vi "Configure Arming (External).vi"(0 "VISA resource name":refnum<visa-resource-name>, 1 "Measurement (0:Frequency)":i32(ring) items=["Frequency", "Frequency Ratio", "Period", "Totalize", "Phase", "Edge Rise Time", "Edge Fall Time", "Positive Pulse Width", "Negative Pulse Width", "Duty Cycle", "Time Interval", "Volt Maximum", "Volt Minimum"], 5 "Start Slope (0:Positive)":i32(ring) items=["Positive", "Negative"], 7 "Stop Type (0:Auto)":i32(ring) items=["Auto", "Positive", "Negative", "Time"], 9 "Stop Time (0.1s)":dbl=0.1 format="%^#_6g", 11 "error in (no error)":errorcluster, 12 "Time Interval Start":T1 {"Start Slope" items=["Positive", "Negative"]; "Start Delay Value" format="%^#_7g"; "Start Delay Type" items=["None", "Time", "Event"]}, 13 "Time Interval Stop":T2 {"Stop Delay Value" format="%^#_7g"; "Stop Delay Type" items=["None", "Time", "Event"]; "Stop Slope" items=["Positive", "Negative"]; "Stop Type" items=["Auto", "External"]}) -> (4 "VISA resource name out":refnum<visa-resource-name>, 15 "error out":errorcluster)   [LabVIEW 2013, in "Counter.lvlib" / "PICOTEST U62XXA series.lvlib"]
doc: "Configures the parameters required for External Arming. This VI should be called after the Configure Measurement VI.\n\n<B>Note:</B>\n\nVolt Peak Measurements <B>does not</B> have External Arming capabilities. Totalize Measurement <B>does not</B> support Auto stop type. The <B>clusters</B> are for Time Interval Measurement only."
uses:
  PICOTEST U62XXA series.lvlib
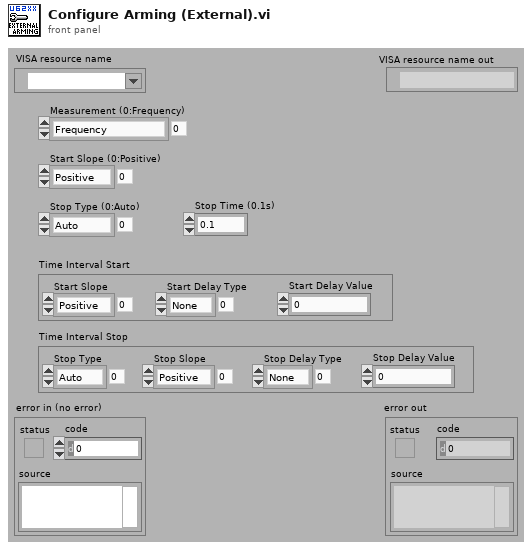
[diagram p1: front panel]
types:
  T1 = cluster{"Start Delay Type":i32, "Start Delay Value":dbl, "Start Slope":i32}
  T2 = cluster{"Stop Type":i32, "Stop Slope":i32, "Stop Delay Type":i32, "Stop Delay Value":dbl}
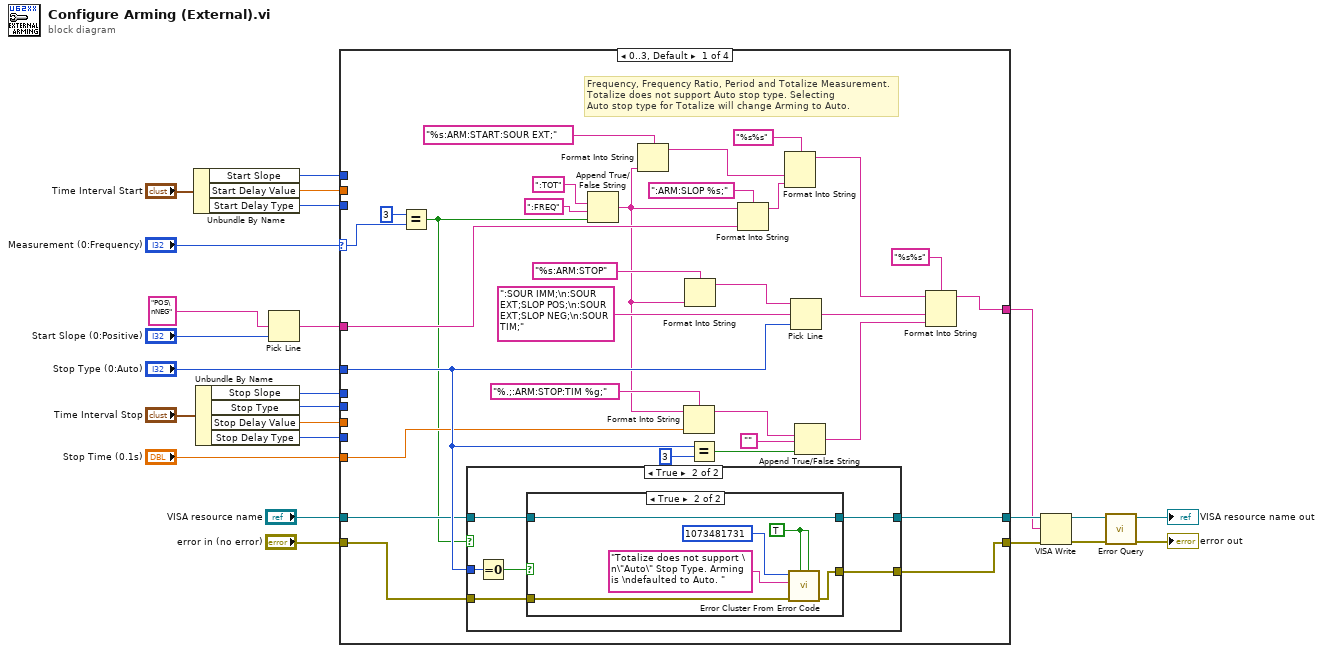
[diagram p0: block diagram]
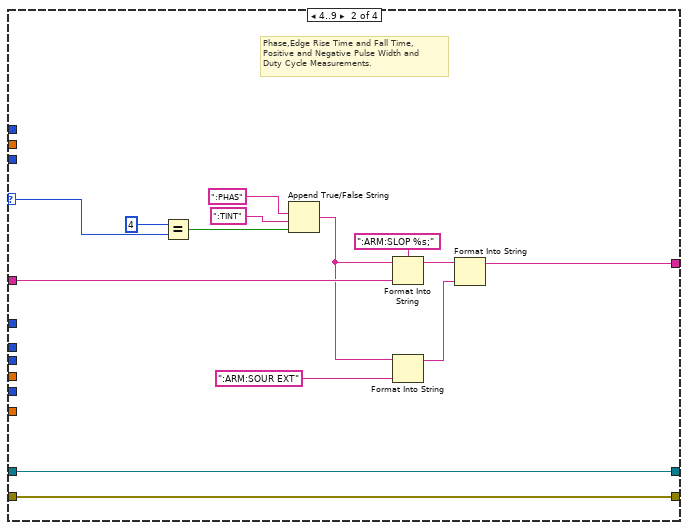
[diagram p4: hidden frame]
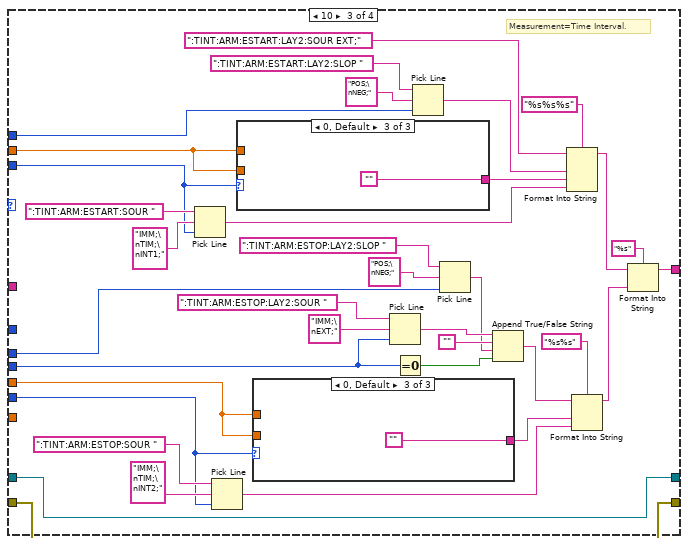
[diagram p5: hidden frame]
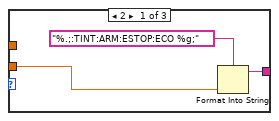
[diagram p6: hidden frame]
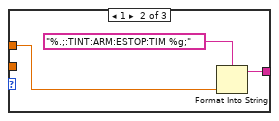
[diagram p7: hidden frame]
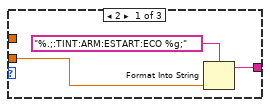
[diagram p8: hidden frame]
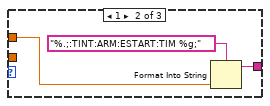
[diagram p9: hidden frame]
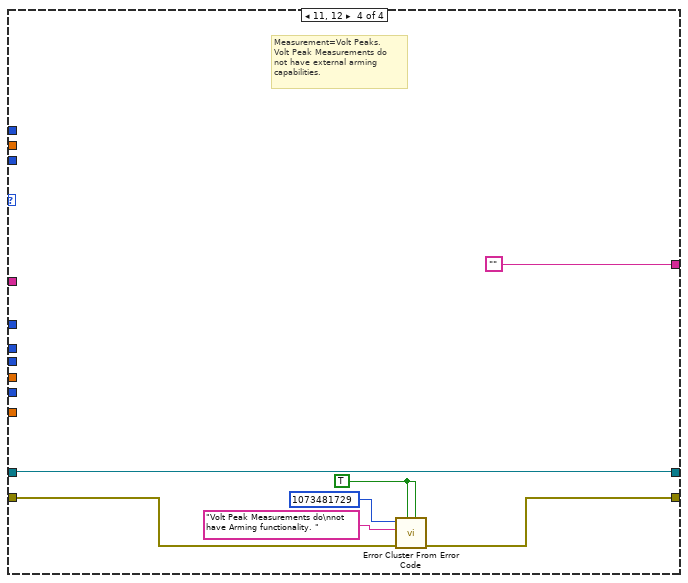
[diagram p10: hidden frame]
diagram:
  n1 = Unbundle By Name("Time Interval Start") -> ("Start Slope"=w13:i32, "Start Delay Value"=w12:dbl, "Start Delay Type"=w11:i32)
  n2 = Unbundle By Name("Time Interval Stop") -> ("Stop Slope"=w9:i32, "Stop Type"=w6:i32, "Stop Delay Value"=w7:dbl, "Stop Delay Type"=w8:i32)
  n3 = Pick Line(multi-line string="POS\nNEG", line index="Start Slope (0:Positive)") -> (output string=w21:string)  [unwired: 1 in]
  n4 = case shown="0..3, Default" "Measurement (0:Frequency)" {
    selector: "Measurement (0:Frequency)" -> [w54 w84 _ _]
    tunnel: w21 -> [w52 w82 _ _]
    tunnel: [w28 w72 w89 ""] -> w1
    tunnel: "Stop Time (0.1s)" -> [w38 _ _ _]
    tunnel: "Stop Type (0:Auto)" -> [w43 _ _ _]
    tunnel: w13 -> [_ _ w112 _]
    tunnel: w12 -> [_ _ w111 _]
    tunnel: w11 -> [_ _ w110 _]
    tunnel: w9 -> [_ _ w103 _]
    tunnel: w6 -> [_ _ w102 _]
    tunnel: w8 -> [_ _ w109 _]
    tunnel: w7 -> [_ _ w108 _]
    tunnel: "VISA resource name" -> [w40 w78 w101 w138]
    tunnel: [w39 w78 w101 w138] -> w4
    tunnel: "error in (no error)" -> [w42 w77 w100 w139]
    tunnel: [w41 w77 w100 w137] -> w2
    frame 0..3, Default {
      # "Frequency, Frequency Ratio, Period and Totalize Measurement. \nTotalize does not support Auto stop type. Selecting\nAuto stop type for Totalize will change Arming to Auto."
      n5 = Equal?(x=3 ("y"), y=w54) -> (x = y?=w37:bool)
      n6 = case shown="True" w37 {
        tunnel: w43 -> [_ w62]
        tunnel: w42 -> [w56 w61]
        tunnel: [w56 w60] -> w41
        tunnel: w40 -> [w57 w59]
        tunnel: [w57 w58] -> w39
        frame False {
        }
        frame True {
          n7 = Equal To 0?(x=w62) -> (x = 0?=w63:bool)
          n8 = case shown="True" w63 {
            tunnel: w61 -> [w65 w68]
            tunnel: [w65 w67] -> w60
            tunnel: w59 -> [w64 w66]
            tunnel: [w64 w66] -> w58
            frame False {
            }
            frame True {
              w69 = TRUE ("is warning? (False)")
              n9 = call <vilib>:"Error Cluster From Error Code.vi"("is warning? (False)"=w69, "show call chain? (False)"=w69, "error in (no error)"=w68, "error message (\"\")"="Totalize does not support \n\"Auto\" Stop Type. Arming is \ndefaulted to Auto. " ("error message (\"\")"), "error code (0)"=1073481731 ("Code")) -> ("error out"=w67:errorcluster)  [unwired: 4 in]
            }
          }
        }
      }
      n10 = Append True/False String(1:w37, 2:":FREQ" ("multi-line string"), 3:":TOT" ("multi-line string")) -> (0:w31:string)  [unwired: 1 in]
      n11 = Format Into String(format string="%s:ARM:START:SOUR EXT;" ("multi-line string"), w31) -> (resulting string=w34:string)  [unwired: 2 in, 1 out]
      n12 = Format Into String(format string="%.;:ARM:STOP:TIM %g;", initial string=w31, w38) -> (resulting string=w47:string)  [unwired: 1 in, 1 out]
      n13 = Format Into String(format string="%s:ARM:STOP" ("multi-line string"), w31) -> (resulting string=w30:string)  [unwired: 2 in, 1 out]
      n14 = Equal?(x=w43, y=3) -> (x = y?=w48:bool)
      n15 = Format Into String(format string=":ARM:SLOP %s;", initial string=w31, w52) -> (resulting string=w33:string)  [unwired: 1 in, 1 out]
      n16 = Format Into String(format string="%s%s", w34, w33) -> (resulting string=w27:string)  [unwired: 2 in, 1 out]
      n17 = Pick Line(string ("")=w30, multi-line string=":SOUR IMM;\n:SOUR EXT;SLOP POS;\n:SOUR EXT;SLOP NEG;\n:SOUR TIM;", line index=w43) -> (output string=w26:string)
      n18 = Append True/False String(1:w48, 2:"", 3:w47) -> (0:w25:string)  [unwired: 1 in]
      n19 = Format Into String(format string="%s%s", initial string=w27, w26, w25) -> (resulting string=w28:string)  [unwired: 1 in, 1 out]
    }
    frame 4..9 {
      # "Phase,Edge Rise Time and Fall Time,\nPositive and Negative Pulse Width and\nDuty Cycle Measurements."
      n20 = Equal?(x=4 ("y"), y=w84) -> (x = y?=w79:bool)
      n21 = Append True/False String(1:w79, 2:":TINT" ("multi-line string"), 3:":PHAS" ("multi-line string")) -> (0:w76:string)  [unwired: 1 in]
      n22 = Format Into String(format string=":ARM:SLOP %s;", initial string=w76, w82) -> (resulting string=w74:string)  [unwired: 1 in, 1 out]
      n23 = Format Into String(initial string=w76, ":ARM:SOUR EXT" ("multi-line string")) -> (resulting string=w73:string)  [unwired: 2 in, 1 out]
      n24 = Format Into String(initial string=w74, w73) -> (resulting string=w72:string)  [unwired: 2 in, 1 out]
    }
    frame 10 {
      # "Measurement=Time Interval."
      n25 = Pick Line(string ("")=":TINT:ARM:ESTART:SOUR ", multi-line string="IMM;\nTIM;\nINT1;", line index=w110) -> (output string=w94:string)
      n26 = Pick Line(string ("")=":TINT:ARM:ESTOP:SOUR ", multi-line string="IMM;\nTIM;\nINT2;", line index=w109) -> (output string=w90:string)
      n27 = case shown="0, Default" w110 {
        tunnel: [w130 w133 ""] -> w95
        tunnel: w111 -> [w129 _ _]
        tunnel: w111 -> [_ w132 _]
        frame 2 {
          n28 = Format Into String(format string="%.;:TINT:ARM:ESTART:ECO %g;", w129) -> (resulting string=w130:string)  [unwired: 2 in, 1 out]
        }
        frame 1 {
          n29 = Format Into String(format string="%.;:TINT:ARM:ESTART:TIM %g;", w132) -> (resulting string=w133:string)  [unwired: 2 in, 1 out]
        }
        frame 0, Default {
        }
      }
      n30 = case shown="0, Default" w109 {
        tunnel: [w123 w126 ""] -> w91
        tunnel: w108 -> [_ w125 _]
        tunnel: w108 -> [w122 _ _]
        frame 2 {
          n31 = Format Into String(format string="%.;:TINT:ARM:ESTOP:ECO %g;", w122) -> (resulting string=w123:string)  [unwired: 2 in, 1 out]
        }
        frame 1 {
          n32 = Format Into String(format string="%.;:TINT:ARM:ESTOP:TIM %g;", w125) -> (resulting string=w126:string)  [unwired: 2 in, 1 out]
        }
        frame 0, Default {
        }
      }
      n33 = Pick Line(string ("")=":TINT:ARM:ESTOP:LAY2:SOUR ", multi-line string="IMM;\nEXT;", line index=w102) -> (output string=w107:string)
      n34 = Equal To 0?(x=w102) -> (x = 0?=w106:bool)
      n35 = Pick Line(string ("")=":TINT:ARM:ESTART:LAY2:SLOP ", multi-line string="POS;\nNEG;", line index=w112) -> (output string=w96:string)
      n36 = Pick Line(string ("")=":TINT:ARM:ESTOP:LAY2:SLOP ", multi-line string="POS;\nNEG;", line index=w103) -> (output string=w104:string)
      n37 = Append True/False String(1:w106, 2:w104, 3:"", 4:w107) -> (0:w92:string)
      n38 = Format Into String(format string="%s%s%s", initial string=":TINT:ARM:ESTART:LAY2:SOUR EXT;", w96, w95, w94) -> (resulting string=w88:string)  [unwired: 1 in, 1 out]
      n39 = Format Into String(format string="%s%s", initial string=w92, w91, w90) -> (resulting string=w87:string)  [unwired: 1 in, 1 out]
      n40 = Format Into String(format string="%s", initial string=w88, w87) -> (resulting string=w89:string)  [unwired: 1 in, 1 out]
    }
    frame 11, 12 {
      w141 = TRUE ("is warning? (False)")
      # "Measurement=Volt Peaks.\nVolt Peak Measurements do\nnot have external arming \ncapabilities."
      n41 = call <vilib>:"Error Cluster From Error Code.vi"("is warning? (False)"=w141, "show call chain? (False)"=w141, "error in (no error)"=w139, "error message (\"\")"="Volt Peak Measurements do\nnot have Arming functionality. " ("error message (\"\")"), "error code (0)"=1073481729 ("Code")) -> ("error out"=w137:errorcluster)  [unwired: 4 in]
    }
  }
  n42 = VISA Write(VISA resource name=w4, write buffer=w1, error in (no error)=w2) -> (VISA resource name out=w20:refnum<visa-resource-name>, error out=w19:errorcluster)  [unwired: 1 out]
  n43 = call "Error Query.vi"("error in (no error)"=w19, "VISA resource name"=w20) -> ("error out"=→"error out":errorcluster, "VISA resource name out"=→"VISA resource name out":refnum<visa-resource-name>)  [unwired: 6 in, 2 out]
